vi "VisionPose.vi"(0 "Lime Vision Target Valid [t-?]":bool, 1 "Lime AprilTag Data [t-?]":dbl[](array[numeric]), 3 "Lemon Vision Target Valid [t-?]":bool, 5 "Lemon AprilTag Data [t-?]":dbl[](array[numeric]), 6 "Odometry Delta X (in) [t0]":dbl, 7 "Vision Trust Threshold (in)":dbl, 8 "Odometry Delta Y (in) [t0]":dbl, 9 "Max Vision X (in)":dbl=200.0, 10 "Using 3D Targeting":bool=TRUE, 11 "Lime Vision Timestamp (ms)":u32, 13 "Lemon Vision Timestamp (ms)":u32) -> (14 "Lime Vision Valid [t-?]":bool, 15 "Combined Vision X (in) [t-?]":dbl, 16 "Combined Vision Y (in) [t-?]":dbl, 17 "Lemon Vision Valid [t-?]":bool, 19 "Lowest Vision Timestamp (ms) [t-?]":u32)   [LabVIEW 2023]
doc: "Calculates the robot pose using the AprilTag data from the LimeLight camera. Also performs additional validation checks to determine if the vision data should be trusted."
uses:
  d330619a-1645-40d1-9d50-519401bd8c1e.vi
  4285d199-8f61-4066-b628-7d31460b52c1.vi
  4345cbd7-6e71-4cf8-9373-c11d187320e6.vi
  bf1fb2dd-70e0-494a-a402-0f0a51a374ae.vi
  9b06592c-c2d2-465c-860e-e540abcedcfa.vi
  4abe6c79-5448-4b86-996e-c08ea5318c24.vi
  57bda909-449e-4d87-9eb9-8530c9f662e1.vi
  95eb604c-32c0-4500-bfee-c4739266980d.vi
  GlobalPoseAndTargeting.vi
  GlobalDriverStationData.vi
  bf2c44f6-4b0d-4fe5-83c9-7a6363c448bc.vi
  4d92e11d-7e53-4506-aad3-8a762df29d8d.vi
panel:
  in  "Limelight pitch(deg)":dbl=40.0
  in  "Limelight z offset(in)":dbl=15.4 format="%#_13g"
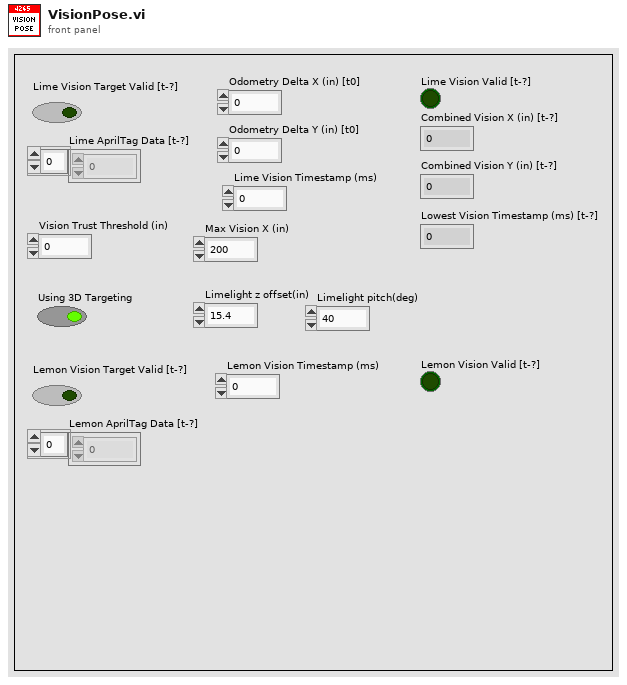
[diagram p1: front panel]
types:
  T1 = typedef "WPI_DriverStationAllianceInfo.ctl" = enum16{"Red", "Blue", "Invalid"}
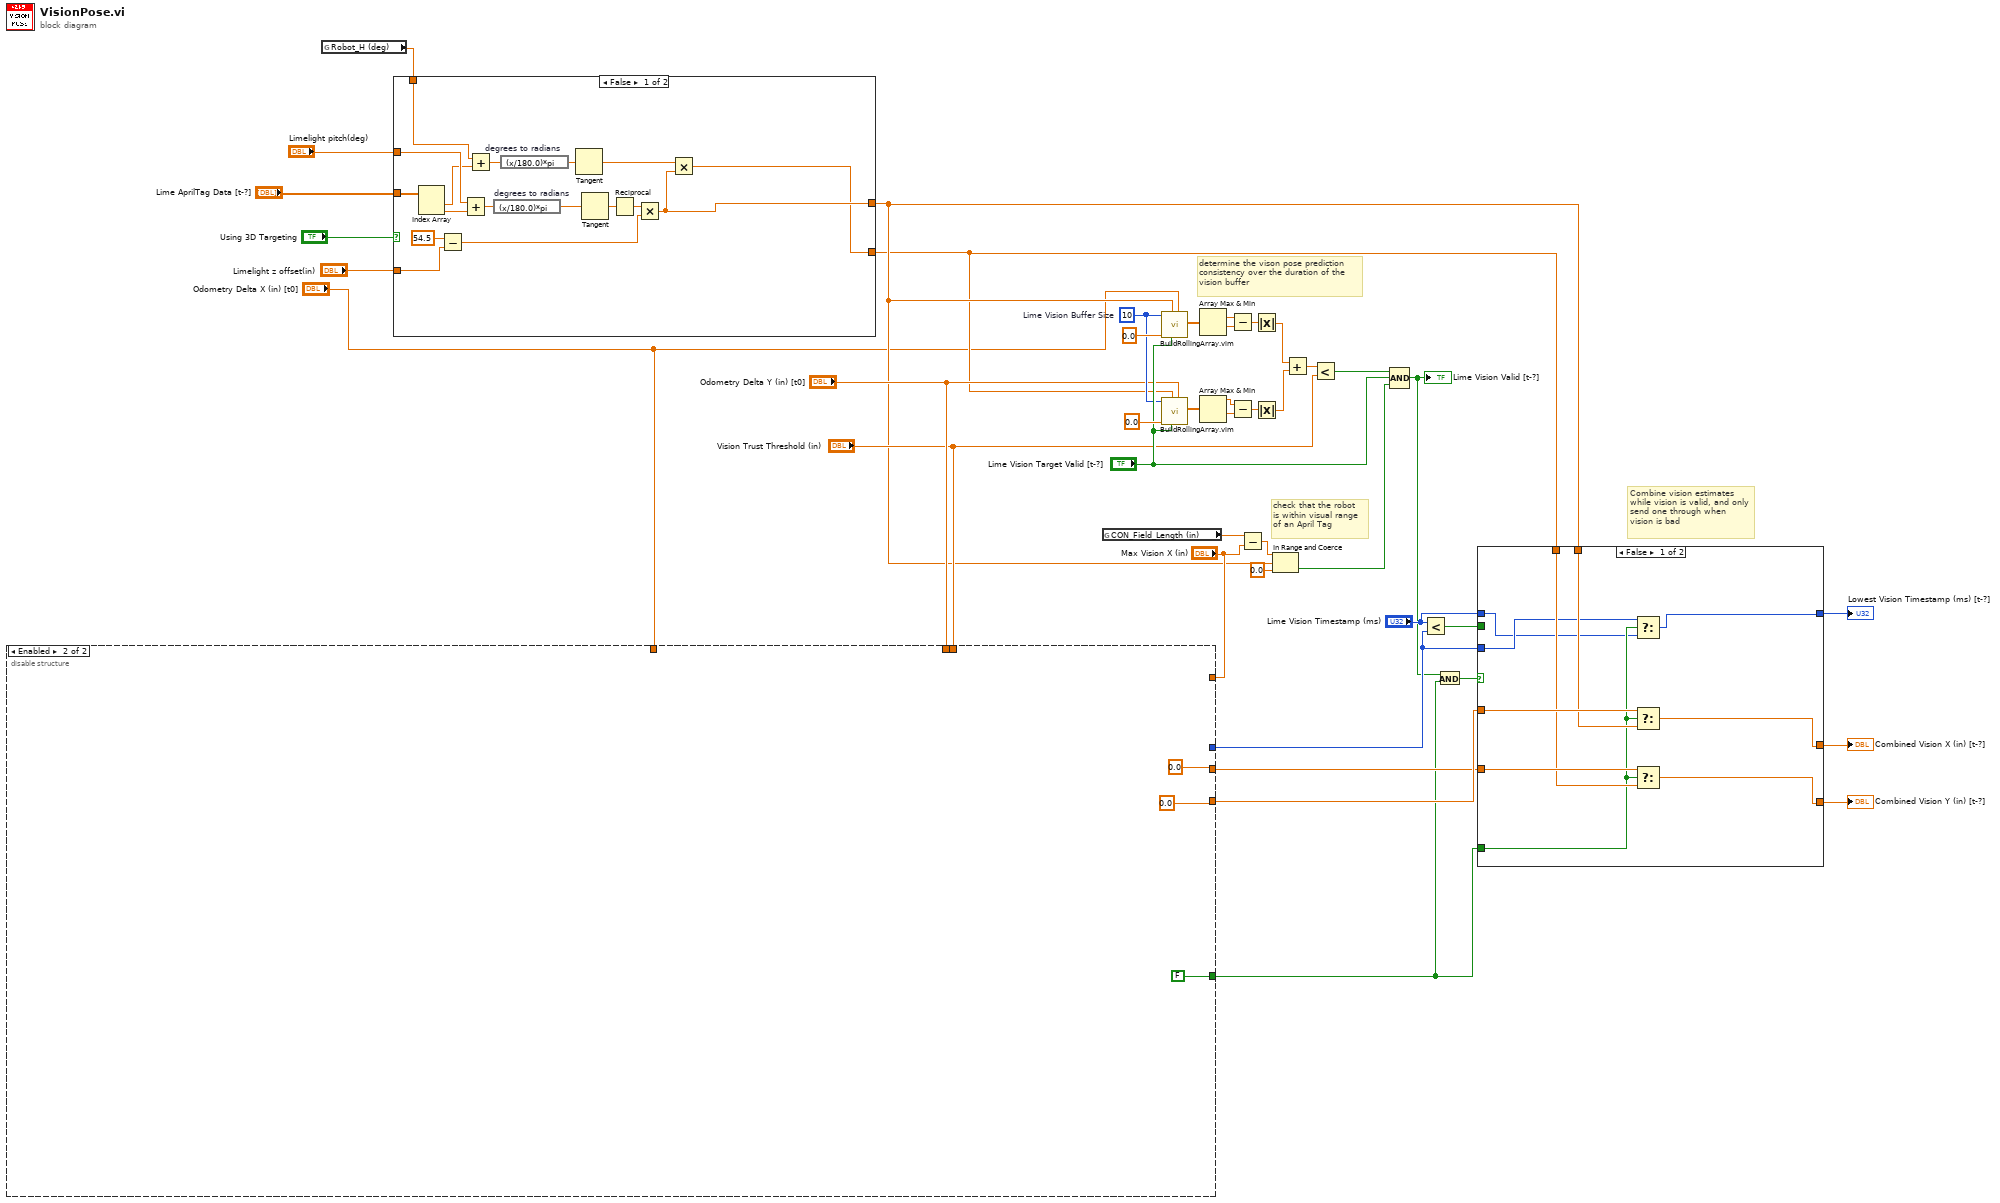
[diagram p0: block diagram]
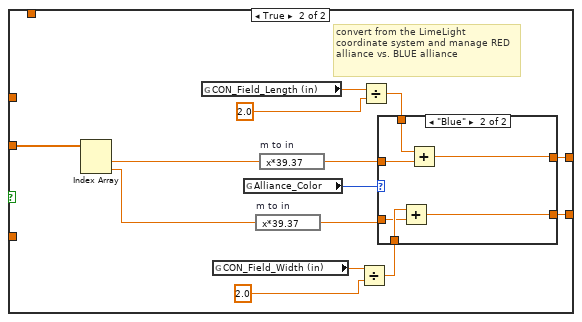
[diagram p2: hidden frame]
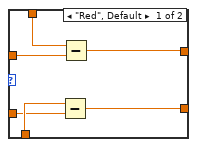
[diagram p3: hidden frame]
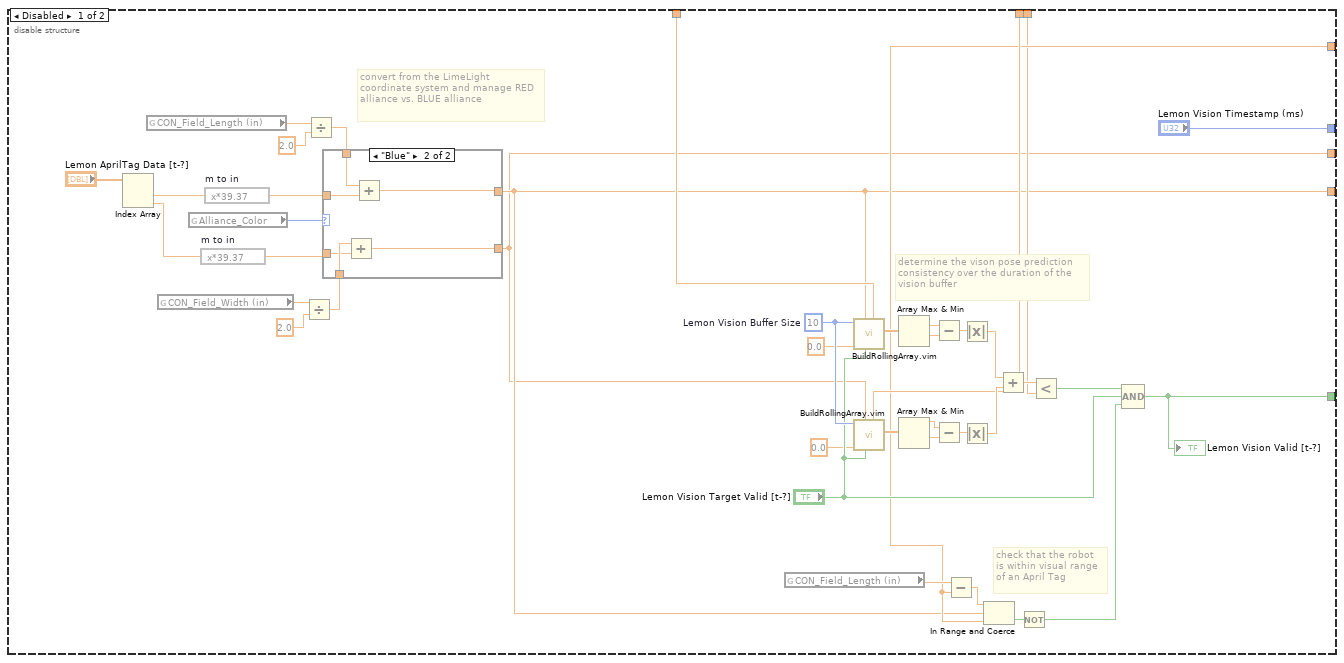
[diagram p4: hidden frame]
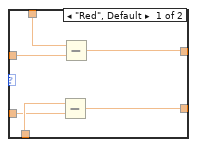
[diagram p5: hidden frame]
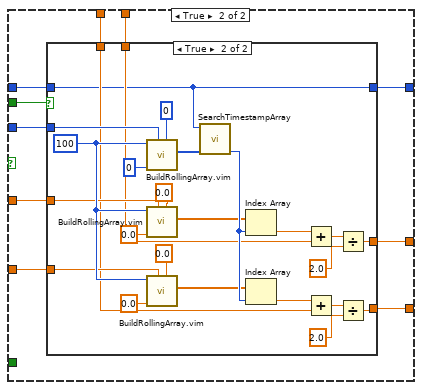
[diagram p6: hidden frame]
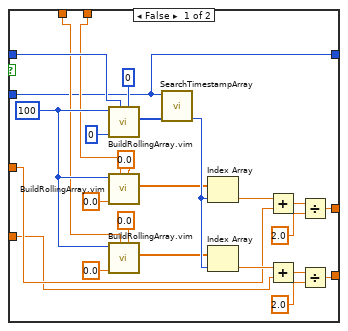
[diagram p7: hidden frame]
diagram:
  w27 = 10  # Lime Vision Buffer Size
  # "Combine vision estimates while vision is valid, and only send one through when vision is bad"
  # "check that the robot\nis within visual range\nof an April Tag"
  # "determine the vison pose prediction\nconsistency over the duration of the\nvision buffer"
  n1 = disable-structure shown="Enabled" {
    disable-tunnel: "Odometry Delta X (in) [t0]" -> [w50 _]
    disable-tunnel: "Odometry Delta Y (in) [t0]" -> [w49 _]
    disable-tunnel: "Max Vision X (in)" -> [w48 _]
    disable-tunnel: "Vision Trust Threshold (in)" -> [w47 _]
    disable-tunnel: ["Lemon Vision Timestamp (ms)" _] -> w19
    disable-tunnel: [w45 0.0] -> w17
    disable-tunnel: [w44 0.0] -> w16
    disable-tunnel: [w43 FALSE] -> w7
    frame Disabled {
      w66 = 10  # Lemon Vision Buffer Size
      # "check that the robot\nis within visual range\nof an April Tag"
      # "convert from the LimeLight\ncoordinate system and manage RED alliance vs. BLUE alliance"
      # "determine the vison pose prediction\nconsistency over the duration of the\nvision buffer"
      n2 = Index Array(array="Lemon AprilTag Data [t-?]") -> (element #1=w68:dbl, element #2=w69:dbl)  [unwired: 2 in]
      n3 = global read "GlobalPoseAndTargeting.vi" "CON_Field_Length (in)"() -> (w71:dbl)
      n4 = global read "GlobalPoseAndTargeting.vi" "CON_Field_Width (in)"() -> (w74:dbl)
      n5 = global read "GlobalDriverStationData.vi" "Alliance_Color"() -> (w70:T1)
      n6 = expression code="x*39.37" "m to in"(w69) -> (w78:dbl)
      n7 = expression code="x*39.37" "m to in"(w68) -> (w77:dbl)
      n8 = Divide(x=w74, y=2.0) -> (x/y=w76:dbl)
      n9 = Divide(x=w71, y=2.0) -> (x/y=w73:dbl)
      n10 = case shown="\"Blue\"" w70 {
        tunnel: w73 -> [w88 w92]
        tunnel: w76 -> [w87 w91]
        tunnel: w78 -> [w86 w90]
        tunnel: w77 -> [w85 w94]
        tunnel: [w84 w93] -> w45
        tunnel: [w83 w89] -> w44
        frame "Red", Default {
          n11 = Subtract(x=w87, y=w86) -> (x-y=w83:dbl)
          n12 = Subtract(x=w88, y=w85) -> (x-y=w84:dbl)
        }
        frame "Blue" {
          n13 = Add(x=w91, y=w90) -> (x+y=w89:dbl)
          n14 = Add(x=w92, y=w94) -> (x+y=w93:dbl)
        }
      }
      n15 = global read "GlobalPoseAndTargeting.vi" "CON_Field_Length (in)"() -> (w81:dbl)
      n16 = call "BuildRollingArray.vim"("Global Additive Update"=w50, "Update?"="Lemon Vision Target Valid [t-?]", "New Value"=w45, "Initial Value"=0.0, "Number of Elements"=w66) -> ("Current Array"=w56:dbl[])  [unwired: 6 in]
      n17 = call "BuildRollingArray.vim"("Global Additive Update"=w49, "Update?"="Lemon Vision Target Valid [t-?]", "New Value"=w44, "Initial Value"=0.0, "Number of Elements"=w66) -> ("Current Array"=w61:dbl[])  [unwired: 6 in]
      n18 = Array Max & Min(array=w56) -> (max value=w57:dbl, min value=w58:dbl)  [unwired: 2 out]
      n19 = Array Max & Min(array=w61) -> (max value=w62:dbl, min value=w60:dbl)  [unwired: 2 out]
      n20 = Subtract(x=w57, y=w58) -> (x-y=w54:dbl)
      n21 = Subtract(x=w62, y=w60) -> (x-y=w59:dbl)
      n22 = Subtract(x=w81, y=w48) -> (x-y=w82:dbl)
      n23 = Absolute Value(x=w54) -> (abs(x)=w55:dbl)
      n24 = Absolute Value(x=w59) -> (abs(x)=w63:dbl)
      n25 = In Range and Coerce(upper limit=w82, x=w45, lower limit=w48) -> (In Range?=w79:bool)  [unwired: 1 out]
      n26 = Add(x=w55, y=w63) -> (x+y=w53:dbl)
      n27 = Not(x=w79) -> (.not. x?=w80:bool)
      n28 = Less?(x=w53, y=w47) -> (x < y?=w64:bool)
      n29 = Compound Arithmetic op=AND(w64, "Lemon Vision Target Valid [t-?]", w80) -> (w43:bool)
      "Lemon Vision Valid [t-?]" <- w43
    }
    frame Enabled {
    }
  }
  n30 = global read "GlobalPoseAndTargeting.vi" "Robot_H (deg)"() -> (w1:dbl)
  n31 = case shown="False" "Using 3D Targeting" {
    tunnel: "Lime AprilTag Data [t-?]" -> [w114 w128]
    tunnel: [w105 w116] -> w15
    tunnel: [w104 w115] -> w14
    tunnel: "Limelight z offset(in)" -> [w109 _]
    tunnel: "Limelight pitch(deg)" -> [w108 _]
    tunnel: w1 -> [w99 _]
    frame False {
      n32 = Index Array(array=w114) -> (element #1=w100:dbl, element #2=w113:dbl)  [unwired: 2 in]
      n33 = Subtract(x=54.5 ("y"), y=w109) -> (x-y=w107:dbl)
      n34 = Add(x=w108, y=w113) -> (x+y=w102:dbl)
      n35 = Add(x=w99, y=w100) -> (x+y=w98:dbl)
      n36 = expression code="(x/180.0)*pi" "degrees to radians"(w102) -> (w103:dbl)
      n37 = expression code="(x/180.0)*pi" "degrees to radians"(w98) -> (w101:dbl)
      n38 = Tangent(1:w101) -> (0:w106:dbl)
      n39 = Tangent(1:w103) -> (0:w112:dbl)
      n40 = Reciprocal(x=w112) -> (1/x=w111:dbl)
      n41 = Multiply(x=w111, y=w107) -> (x*y=w105:dbl)
      n42 = Multiply(x=w106, y=w105) -> (x*y=w104:dbl)
    }
    frame True {
      # "convert from the LimeLight\ncoordinate system and manage RED alliance vs. BLUE alliance"
      n43 = Index Array(array=w128) -> (element #1=w127:dbl, element #2=w126:dbl)  [unwired: 2 in]
      n44 = global read "GlobalPoseAndTargeting.vi" "CON_Field_Length (in)"() -> (w124:dbl)
      n45 = global read "GlobalPoseAndTargeting.vi" "CON_Field_Width (in)"() -> (w121:dbl)
      n46 = global read "GlobalDriverStationData.vi" "Alliance_Color"() -> (w125:T1)
      n47 = expression code="x*39.37" "m to in"(w126) -> (w117:dbl)
      n48 = expression code="x*39.37" "m to in"(w127) -> (w118:dbl)
      n49 = Divide(x=w121, y=2.0) -> (x/y=w119:dbl)
      n50 = Divide(x=w124, y=2.0) -> (x/y=w122:dbl)
      n51 = case shown="\"Blue\"" w125 {
        tunnel: w122 -> [w134 w138]
        tunnel: w119 -> [w133 w137]
        tunnel: w117 -> [w132 w136]
        tunnel: w118 -> [w131 w140]
        tunnel: [w130 w139] -> w116
        tunnel: [w129 w135] -> w115
        frame "Red", Default {
          n52 = Subtract(x=w133, y=w132) -> (x-y=w129:dbl)
          n53 = Subtract(x=w134, y=w131) -> (x-y=w130:dbl)
        }
        frame "Blue" {
          n54 = Add(x=w137, y=w136) -> (x+y=w135:dbl)
          n55 = Add(x=w138, y=w140) -> (x+y=w139:dbl)
        }
      }
    }
  }
  n56 = global read "GlobalPoseAndTargeting.vi" "CON_Field_Length (in)"() -> (w24:dbl)
  n57 = call "BuildRollingArray.vim"("Global Additive Update"="Odometry Delta X (in) [t0]", "Update?"="Lime Vision Target Valid [t-?]", "New Value"=w15, "Initial Value"=0.0, "Number of Elements"=w27) -> ("Current Array"=w37:dbl[])  [unwired: 6 in]
  n58 = call "BuildRollingArray.vim"("Global Additive Update"="Odometry Delta Y (in) [t0]", "Update?"="Lime Vision Target Valid [t-?]", "New Value"=w14, "Initial Value"=0.0, "Number of Elements"=w27) -> ("Current Array"=w32:dbl[])  [unwired: 6 in]
  n59 = Array Max & Min(array=w37) -> (max value=w36:dbl, min value=w35:dbl)  [unwired: 2 out]
  n60 = Array Max & Min(array=w32) -> (max value=w31:dbl, min value=w33:dbl)  [unwired: 2 out]
  n61 = Subtract(x=w36, y=w35) -> (x-y=w39:dbl)
  n62 = Subtract(x=w31, y=w33) -> (x-y=w34:dbl)
  n63 = Subtract(x=w24, y="Max Vision X (in)") -> (x-y=w23:dbl)
  n64 = Absolute Value(x=w39) -> (abs(x)=w38:dbl)
  n65 = Absolute Value(x=w34) -> (abs(x)=w30:dbl)
  n66 = In Range and Coerce(upper limit=w23, x=w15, lower limit=0.0) -> (In Range?=w25:bool)  [unwired: 1 out]
  n67 = Add(x=w38, y=w30) -> (x+y=w40:dbl)
  n68 = Less?(x=w40, y="Vision Trust Threshold (in)") -> (x < y?=w29:bool)
  n69 = Compound Arithmetic op=AND(w29, "Lime Vision Target Valid [t-?]", w25) -> (w9:bool)
  "Lime Vision Valid [t-?]" <- w9
  n70 = Less?(x="Lime Vision Timestamp (ms)", y=w19) -> (x < y?=w13:bool)
  n71 = And(x=w9, y=w7) -> (x .and. y?=w8:bool)
  n72 = case shown="False" w8 {
    tunnel: w19 -> [w143 w160]
    tunnel: "Lime Vision Timestamp (ms)" -> [w141 w159]
    tunnel: w17 -> [w150 w158]
    tunnel: w16 -> [w149 w157]
    tunnel: w15 -> [w147 w156]
    tunnel: w14 -> [w148 w155]
    tunnel: w13 -> [_ w154]
    tunnel: [w146 w153] -> w12
    tunnel: [w145 w152] -> w11
    tunnel: [w142 w151] -> w10
    tunnel: w7 -> [w144 _]
    frame False {
      n73 = Select(t=w143, s=w144, f=w141) -> (s? t:f=w142:u32)
      n74 = Select(t=w150, s=w144, f=w147) -> (s? t:f=w146:dbl)
      n75 = Select(t=w149, s=w144, f=w148) -> (s? t:f=w145:dbl)
    }
    frame True {
      n76 = case shown="True" w154 {
        tunnel: w160 -> [w161 w210]
        tunnel: w159 -> [w168 w186]
        tunnel: w158 -> [w165 w203]
        tunnel: w157 -> [w164 w202]
        tunnel: w156 -> [w166 w194]
        tunnel: w155 -> [w167 w193]
        tunnel: [w163 w188] -> w153
        tunnel: [w162 w187] -> w152
        tunnel: [w161 w186] -> w151
        frame False {
          w182 = 100 ("Number of Elements")
          n77 = call "BuildRollingArray.vim"("Global Additive Update"=0, "New Value"=w168, "Initial Value"=0, "Number of Elements"=w182) -> ("Current Array"=w184:u32[])  [unwired: 7 in]
          n78 = call "BuildRollingArray.vim"("Global Additive Update"=0.0, "New Value"=w166, "Initial Value"=0.0, "Number of Elements"=w182) -> ("Current Array"=w176:dbl[])  [unwired: 7 in]
          n79 = call "BuildRollingArray.vim"("Global Additive Update"=0.0, "New Value"=w167, "Initial Value"=0.0, "Number of Elements"=w182) -> ("Current Array"=w175:dbl[])  [unwired: 7 in]
          n80 = call "SearchTimestampArray.vi"("Timestamp Array"=w184, "Search Timestamp"=w161) -> ("Closest Index"=w177:i32)  [unwired: 8 in, 1 out]
          n81 = Index Array(array=w176, index=w177) -> (element=w173:dbl)
          n82 = Index Array(array=w175, index=w177) -> (element=w174:dbl)
          n83 = Add(x=w173, y=w165) -> (x+y=w172:dbl)
          n84 = Add(x=w174, y=w164) -> (x+y=w169:dbl)
          n85 = Divide(x=w172, y=2.0) -> (x/y=w163:dbl)
          n86 = Divide(x=w169, y=2.0) -> (x/y=w162:dbl)
        }
        frame True {
          w206 = 100 ("Number of Elements")
          n87 = call "BuildRollingArray.vim"("Global Additive Update"=0, "New Value"=w210, "Initial Value"=0, "Number of Elements"=w206) -> ("Current Array"=w208:u32[])  [unwired: 7 in]
          n88 = call "BuildRollingArray.vim"("Global Additive Update"=0.0, "New Value"=w203, "Initial Value"=0.0, "Number of Elements"=w206) -> ("Current Array"=w198:dbl[])  [unwired: 7 in]
          n89 = call "BuildRollingArray.vim"("Global Additive Update"=0.0, "New Value"=w202, "Initial Value"=0.0, "Number of Elements"=w206) -> ("Current Array"=w197:dbl[])  [unwired: 7 in]
          n90 = call "SearchTimestampArray.vi"("Timestamp Array"=w208, "Search Timestamp"=w186) -> ("Closest Index"=w199:i32)  [unwired: 8 in, 1 out]
          n91 = Index Array(array=w198, index=w199) -> (element=w195:dbl)
          n92 = Index Array(array=w197, index=w199) -> (element=w196:dbl)
          n93 = Add(x=w195, y=w194) -> (x+y=w192:dbl)
          n94 = Add(x=w196, y=w193) -> (x+y=w189:dbl)
          n95 = Divide(x=w192, y=2.0) -> (x/y=w188:dbl)
          n96 = Divide(x=w189, y=2.0) -> (x/y=w187:dbl)
        }
      }
    }
  }
  "Combined Vision X (in) [t-?]" <- w12
  "Combined Vision Y (in) [t-?]" <- w11
  "Lowest Vision Timestamp (ms) [t-?]" <- w10
